vi "Create.vi"(7 "Password Encoder (Basic)":refnum<class "Password Encoder.lvclass">, 8 "error in (no error)":errorcluster, 11 "User Init Info":T1) -> (0 "error out":errorcluster, 3 "TestUser out":refnum<class "TestUser.lvclass">)   [LabVIEW 2020, in "TestUser.lvclass"]
uses:
  TestUser.lvclass
  lv-http-server/HTTP Server/Password Encoder/Password Encoder.lvclass
  lv-http-server/HTTP Server/BasicPasswordEncoder/BasicPasswordEncoder.lvclass
  C:/Program Files (x86)/National Instruments/LabVIEW 2020/vi.lib/IlluminatedG/IG HTTP Server/HTTP Server/Password Encoder/Password Encoder.lvclass
  User Init Info.ctl
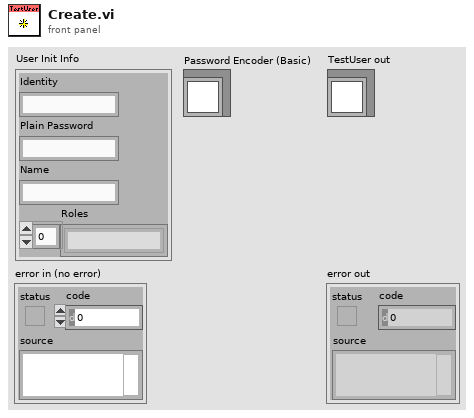
[diagram p1: front panel]
types:
  T1 = typedef "TestUser.lvclass/User Init Info.ctl" = cluster{"Identity":string, "Plain Password":string, "Name":string, "Roles":string[]}
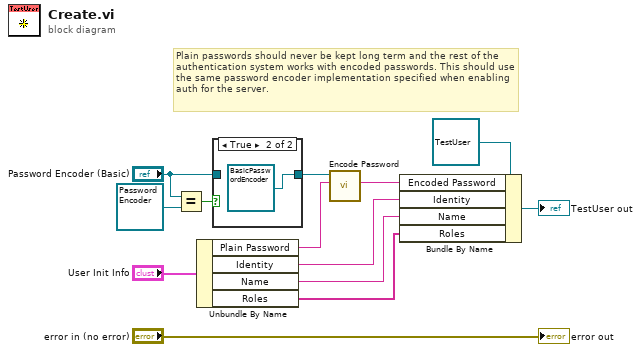
[diagram p0: block diagram]
diagram:
  # "Plain passwords should never be kept long term and the rest of the authentication system works with encoded passwords. This should use the same password encoder implementation specified when enabling auth for the server."
  n1 = Equal?(x="Password Encoder (Basic)", y=refnum<class "Password Encoder.lvclass"> refnum) -> (x = y?=w10:bool)
  n2 = Unbundle By Name("User Init Info") -> ("Plain Password"=w6:string, "Identity"=w3:string, "Name"=w2:string, "Roles"=w1:string[])
  n3 = case shown="True" w10 {
    tunnel: "Password Encoder (Basic)" -> [w14 _]
    tunnel: [w14 refnum<class "BasicPasswordEncoder.lvclass"> refnum ("HTTP Server.lvlib:BasicPasswordEncoder.lvclass")] -> w8
    frame False {
    }
    frame True {
    }
  }
  n4 = call-dynamic "Encode Password.vi"("Plain Password"=w6, "Password Encoder in"=w8) -> ("Encoded Password"=w4:string)  [unwired: 7 in, 2 out]
  n5 = Bundle By Name(cluster=refnum<class "TestUser.lvclass"> refnum ("TestUser in"), "Encoded Password"=w4, "Identity"=w3, "Name"=w2, "Roles"=w1) -> (→"TestUser out":refnum<class "TestUser.lvclass">)
  "error out" <- "error in (no error)"
